vi "Start Async Processing.vi"(7 "Client URI":refnum<class "URI.lvclass">, 8 "error in (no error)":errorcluster, 9 "Secure":bool, 10 "TCP":refnum<k5>, 11 "Server in":refnum<class "Server.lvclass">) -> (0 "error out":errorcluster, 3 "Server out":refnum<class "Server.lvclass">)   [LabVIEW 2020, in "HTTP Server.lvlib" / "Server.lvclass"]
uses:
  Server.lvclass
  Server.lvclass/Server.ctl
  Process Async.vi
  lv-uri/URI/URI/URI.lvclass
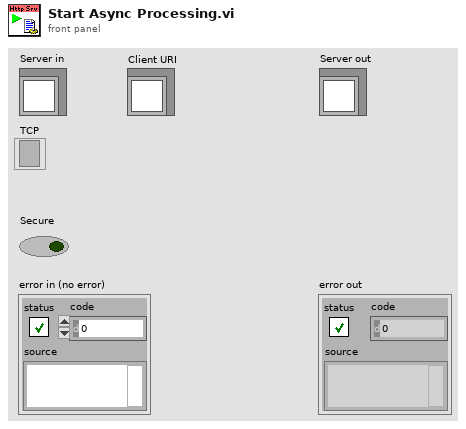
[diagram p1: front panel]
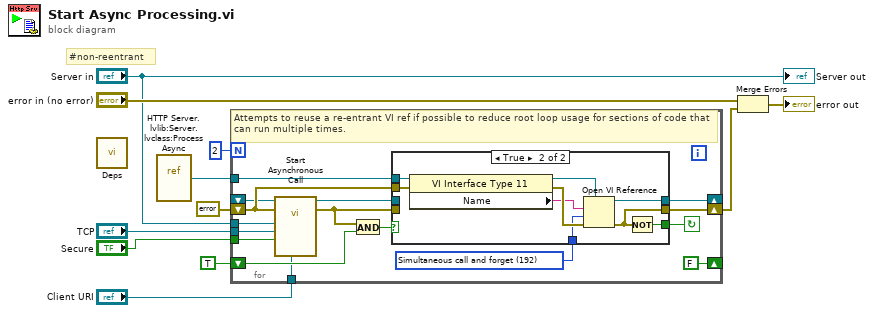
[diagram p0: block diagram]
diagram:
  # "#non-reentrant"
  n1 = call "Deps.vi"() -> ()  [unwired: 12 in]
  n2 = vi-ref "HTTP Server.lvlib:Server.lvclass:Process Async.vi"() -> (w4:refnum<vi>)
  n3 = for {
    N: 2 -> [_]
    tunnel: w4 -> [w26]
    shift-right: [w25] -> _
    shift-left: _ -> [w24]
    shift-right: [w22] -> w3
    shift-left: errorcluster {"status"=FALSE, "code"=0, "source"=""} ("error constant") -> [w27]
    shift-right: [FALSE] -> _
    shift-left: TRUE -> [w19]
    tunnel: "Server in" -> [w15]
    tunnel: "TCP" -> [w14]
    tunnel: "Secure" -> [w13]
    tunnel: "Client URI" -> [w12]
    stop <- w18 continue-if-true
    w16 = 192 items=["Record modifications"=1, "Open templates for editing"=2, "Prompt user to save"=4, "Prepare for reentrant run"=8, "Prompt to find missing subVIs"=16, "Hide loading dialog box"=32, "Enable simultaneous calls"=64, "Prepare to call and forget"=128, "Simultaneous call and forget"=192, "Prepare to call and collect"=256, "Simultaneous call and collect"=320]
    # "Attempts to reuse a re-entrant VI ref if possible to reduce root loop usage for sections of code that can run multiple times."
    n4 = call-by-ref "Start Asynchronous Call"(reference=w24, error in=w27, "Client URI"=w12, "Secure"=w13, "TCP"=w14, "Server in"=w15) -> (reference out=w23:refnum<vi>, error out=w21:errorcluster)  [unwired: 8 in]
    n5 = And(x=w21, y=w19) -> (x .and. y?=w20:bool)
    n6 = case shown="True" w20 {
      tunnel: w26 -> [_ w37]
      tunnel: w16 -> [_ w35]
      tunnel: [w29 w33] -> w25
      tunnel: w23 -> [w29 _]
      tunnel: [w28 w31] -> w22
      tunnel: w21 -> [w28 _]
      tunnel: w27 -> [_ w32]
      tunnel: [_ w30] -> w18
      frame False {
      }
      frame True {
        n7 = property class="VI Interface Type 11"(reference=w37, error in=w32) -> (reference out=w34:refnum<vi>, error out=w38:errorcluster, "Name"=w36:string)
        n8 = Open VI Reference(type specifier VI Refnum (for type only)=w34, vi path=w36, options=w35, error in (no error)=w38) -> (vi reference=w33:refnum<vi>, error out=w31:errorcluster)  [unwired: 2 in]
        n9 = Not(x=w31) -> (.not. x?=w30:bool)
      }
    }
  }
  n10 = Merge Errors("error in (no error)", w3) -> (→"error out":errorcluster)
  "Server out" <- "Server in"
